vi "IC_ImageActiveBuffer_IMAQ.vi"(0 "ICImagingControl In":refnum<k7>, 1 "BorderSize":i32=3, 2 "Error In (no error)":errorcluster) -> (3 "ICImagingControl Out":refnum<k7>, 4 "Image Out":T1, 5 "SampleStartTime":dbl, 6 "Error Out":errorcluster)   [LabVIEW 2020]
uses:
  <vilib>/vision/Image Controls.llb/IMAQ Image.ctl
  IC LabVIEW Extension 2.dll
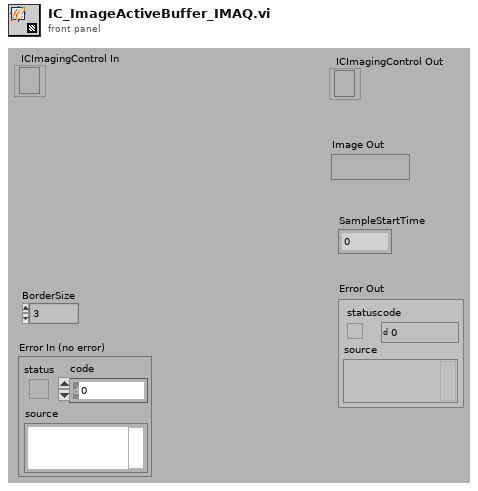
[diagram p1: front panel]
types:
  T1 = typedef "IMAQ Image.ctl" = refnum<image>
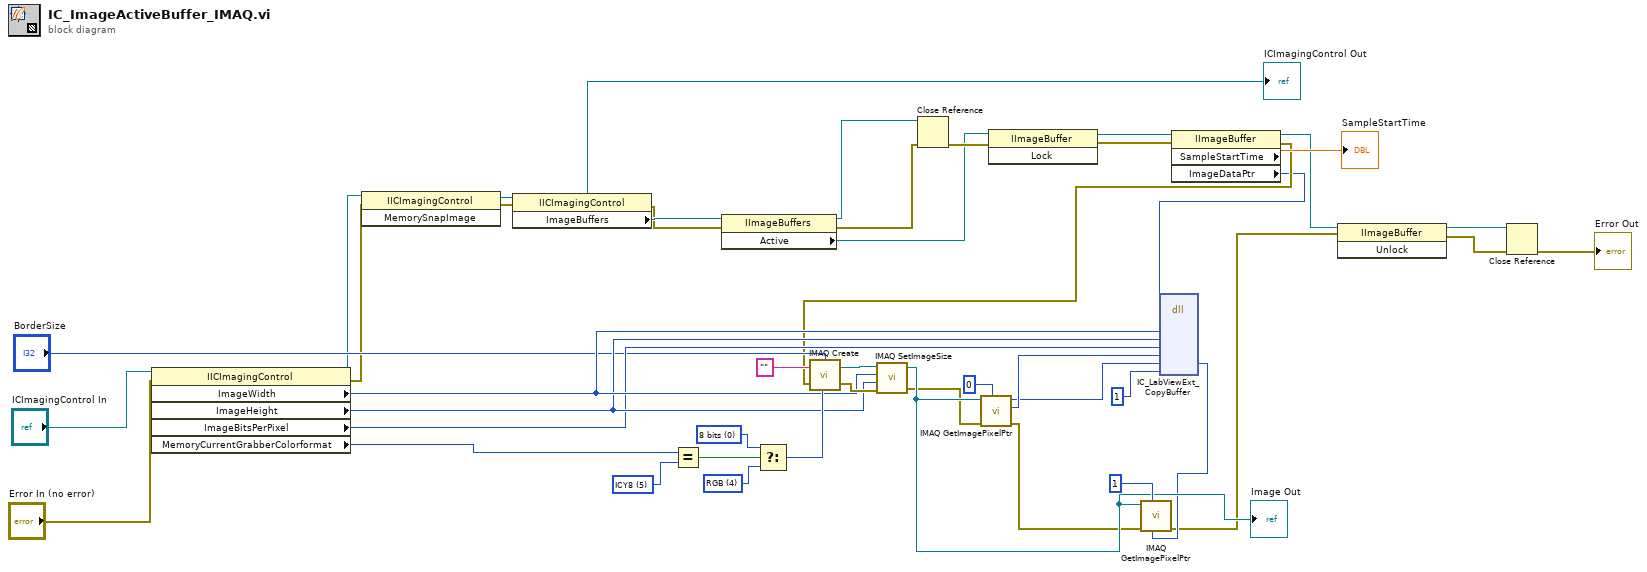
[diagram p0: block diagram]
diagram:
  w32 = 5 items=["ICRGB32"=1, "ICRGB24"=2, "ICRGB565"=3, "ICRGB555"=4, "ICY8"=5, "ICUYVY"=6] ("MemoryCurrentGrabberColorformat")
  w33 = u32 4 items=["8 bits", "16 bits", "Float", "Complex", "RGB", "HSL"] ("Image Type")
  w34 = u32 0 items=["8 bits", "16 bits", "Float", "Complex", "RGB", "HSL"] ("Image Type")
  n1 = property class="IICImagingControl"(reference="ICImagingControl In", error in="Error In (no error)") -> (reference out=w5:refnum<k7>, error out=w4:errorcluster, "ImageWidth"=w31:i32, "ImageHeight"=w30:i32, "ImageBitsPerPixel"=w29:i32, "MemoryCurrentGrabberColorformat"=w41:i32)
  n2 = invoke class="IICImagingControl" method="MemorySnapImage"(reference=w5, error in=w4) -> (reference out=w20:refnum<k7>, error out=w3:errorcluster)  [unwired: 1 in, 1 out]
  n3 = property class="IICImagingControl"(reference=w20, error in=w3) -> (reference out=→"ICImagingControl Out":refnum<k7>, error out=w2:errorcluster, "ImageBuffers"=w23:refnum<k7>)
  n4 = Equal?(x=w41, y=w32) -> (x = y?=w40:bool)
  n5 = property class="IImageBuffers"(reference=w23, error in=w2) -> (reference out=w6:refnum<k7>, error out=w1:errorcluster, "Active"=w7:refnum<k7>)
  n6 = Select(t=w34, s=w40, f=w33) -> (s? t:f=w39:u32)
  n7 = Close Reference(reference=w6, error in (no error)=w1) -> (error out=w10:errorcluster)
  n8 = invoke class="IImageBuffer" method="Lock"(reference=w7, error in=w10) -> (reference out=w8:refnum<k7>, error out=w9:errorcluster)  [unwired: 1 in, 1 out]
  n9 = property class="IImageBuffer"(reference=w8, error in=w9) -> (reference out=w12:refnum<k7>, error out=w13:errorcluster, "SampleStartTime"=→"SampleStartTime":dbl, "ImageDataPtr"=w11:i32)
  n10 = call "IMAQ Create"("Border Size"="BorderSize", "Image Name"="", "Image Type"=w39, "error in (no error)"=w13) -> ("New Image"=w44:T1, "error out"=w38:errorcluster)  [unwired: 1 in]
  n11 = call "IMAQ SetImageSize"("error in (no error)"=w38, "Y Resolution"=w30, "X Resolution"=w31, "Image"=w44) -> ("error out"=w37:errorcluster, "Image Out"=w42:T1)  [unwired: 1 in]
  "Image Out" <- w42
  n12 = call "IMAQ GetImagePixelPtr"("Function"=0, "error in (no error)"=w37, "Image"=w42) -> ("error out"=w36:errorcluster, "LineWidth(Pixels)"=w28:i32, "Pixel Pointer out"=w27:u64)  [unwired: 3 in, 3 out]
  n13 = dll-call lib="C:/data/documents/Fritz-Haber-Institut/Github/ARPEScontrol/subvi/IC/IC LabVIEW Extension 2.dll" fn="IC_LabViewExt_CopyBuffer"("data"=w11, "width"=w31, "height"=w30, "bpp"=w29, "imaq_width"=w28, "imaq_ptr"=w27, "bFlip"=1) -> ("imaq_ptr"=w25:u32)  [unwired: 10 in, 2 out]
  n14 = call "IMAQ GetImagePixelPtr"("Pixel Pointer in"=w25, "Function"=1, "error in (no error)"=w36, "Image"=w42) -> ("error out"=w17:errorcluster)  [unwired: 2 in, 5 out]
  n15 = invoke class="IImageBuffer" method="Unlock"(reference=w12, error in=w17) -> (reference out=w16:refnum<k7>, error out=w15:errorcluster)  [unwired: 1 in, 1 out]
  n16 = Close Reference(reference=w16, error in (no error)=w15) -> (error out=→"Error Out":errorcluster)
